vi "LAB conversion.vi"() -> ()   [LabVIEW 2010]
uses:
  <vilib>/vision/NI_Vision_Development_Module.lvlib
panel:
  out "B":dbl=-47.709583897064704
  out "A":dbl=19.427879668908936
  out "L":dbl=23.243665959549205
  in  "Blue value":u8=128
  in  "Green value":u8=50
  in  "Red value":u8=5
  out "Blue or Luma or Val or Inten or Z or b*value":dbl=-41.32403464435932 format="%.6f"
  out "Green or Sat or Y or a* value":dbl=-1.6051565900875864 format="%.6f"
  out "Red or Hue or X or L* value":dbl=126.40768607184717 format="%.6f"
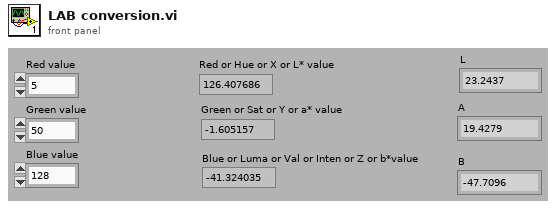
[diagram p1: front panel]
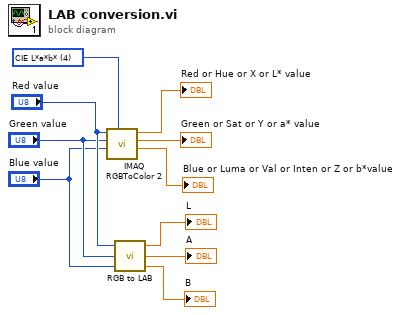
[diagram p0: block diagram]
diagram:
  w10 = u16 4 items=["RGB", "HSL", "HSV", "HSI", "CIE L*a*b*", "CIE XYZ"] ("Color Mode")
  n1 = call "IMAQ RGBToColor 2"("Color Mode"=w10, "Blue value"="Blue value", "Green value"="Green value", "Red value"="Red value") -> ("Blue or Luma or Val or Inten or Z or b*value"=→"Blue or Luma or Val or Inten or Z or b*value":dbl, "Green or Sat or Y or a* value"=→"Green or Sat or Y or a* value":dbl, "Red or Hue or X or L* value"=→"Red or Hue or X or L* value":dbl)  [unwired: 4 in, 1 out]
  n2 = call "RGB to LAB.vi"("Blue"="Blue value", "Green"="Green value", "Red"="Red value") -> ("B"=→"B":dbl, "A"=→"A":dbl, "L"=→"L":dbl)
